vi "DAQNI_task_thermocouple.vi"() -> ()   [LabVIEW 2020]
uses:
  <vilib>/DAQmx/read.llb/DAQmx Read (Analog DBL 1Chan 1Samp).vi
  <vilib>/DAQmx/miscellaneous.llb/DAQmx Fill In Error Info.vi
panel:
  out "s? t:f":string
  out "Threshold exceeded?":bool
  in  "max temp":dbl
  out "error out":errorcluster
  out "current temp (deg C)":dbl format="%0.2f"
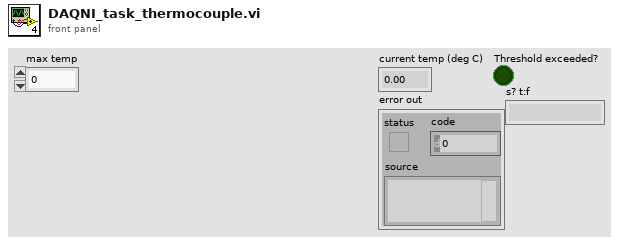
[diagram p1: front panel]
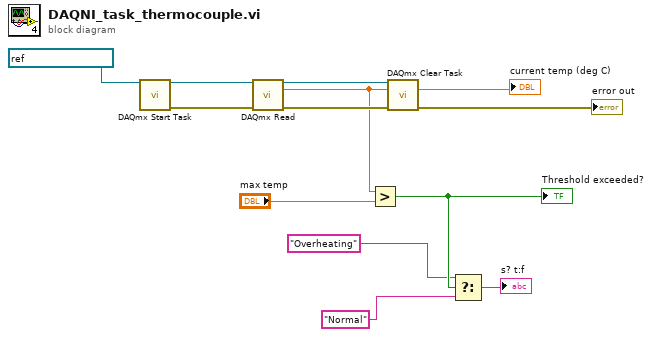
[diagram p0: block diagram]
diagram:
  n1 = call <vilib>:"DAQmx Start Task.vi"("task/channels in"=refnum<k21> "Thermocouple") -> ("task out"=w11:refnum<k21>, "error out"=w9:errorcluster)  [unwired: 13 in]
  n2 = call-poly <vilib>:"DAQmx Read.vi"("task/channels in"=w11, "error in"=w9) -> ("task out"=w10:refnum<k21>, "data"=w6:dbl, "error out"=w8:errorcluster)  [unwired: 11 in]
  "current temp (deg C)" <- w6
  n3 = Greater?(x=w6, y="max temp") -> (0:w4:bool)
  "Threshold exceeded?" <- w4
  n4 = call <vilib>:"DAQmx Clear Task.vi"("task in"=w10, "error in"=w8) -> ("error out"=→"error out":errorcluster)  [unwired: 13 in]
  n5 = Select(t="Overheating", s=w4, f="Normal") -> (s? t:f=→"s? t:f":string)
